vi "Illuminance Correction.vi"(8 "error in (no error)":errorcluster, 11 "Refnum in":T1) -> (0 "error out":errorcluster, 3 "Refnum out":T1)   [LabVIEW 2015]
uses:
  <vilib>/vision/Image Controls.llb/IMAQ Image.ctl
  <vilib>/vision/NI_Vision_Development_Module.lvlib
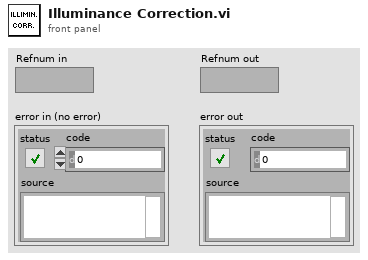
[diagram p1: front panel]
types:
  T1 = typedef "IMAQ Image.ctl" = refnum<image>
  T2 = enum32{"Linear", "Log", "Exp", "Square", "Square root", "Power X", "Power 1/X"}
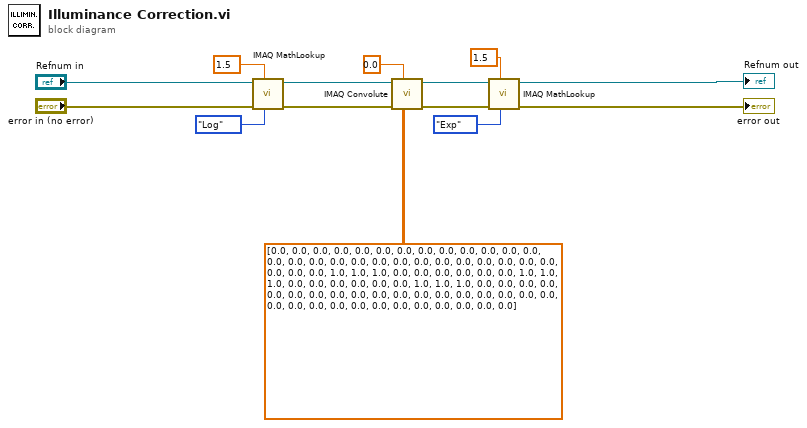
[diagram p0: block diagram]
diagram:
  n1 = call "IMAQ MathLookup"("Operator"=T2."Log", "X Value"=sgl 1.5, "error in (no error)"="error in (no error)", "Image Src"="Refnum in") -> ("error out"=w5:errorcluster, "Image Dst Out"=w7:T1)  [unwired: 3 in, 3 out]
  n2 = call "IMAQ Convolute"("Kernel"=sgl[][] [[0.0, 0.0, 0.0, 0.0, 0.0, 0.0, 0.0, 0.0, 0.0], [0.0, 0.0, 0.0, 0.0, 0.0, 0.0, 0.0, 0.0, 0.0], [0.0, 0.0, 0.0, 0.0, 0.0, 0.0, 0.0, 0.0, 0.0], [0.0, 0.0, 0.0, 1.0, 1.0, 1.0, 0.0, 0.0, 0.0], [0.0, 0.0, 0.0, 1.0, 1.0, 1.0, 0.0, 0.0, 0.0], [0.0, 0.0, 0.0, 1.0, 1.0, 1.0, 0.0, 0.0, 0.0], [0.0, 0.0, 0.0, 0.0, 0.0, 0.0, 0.0, 0.0, 0.0], [0.0, 0.0, 0.0, 0.0, 0.0, 0.0, 0.0, 0.0, 0.0], [0.0, 0.0, 0.0, 0.0, 0.0, 0.0, 0.0, 0.0, 0.0]], "Divider (kernel sum)"=sgl 0.0 ("Divider"), "error in (no error)"=w5, "Image Src"=w7) -> ("error out"=w8:errorcluster, "Image Dst Out"=w12:T1)  [unwired: 3 in, 3 out]
  n3 = call "IMAQ MathLookup"("Operator"=T2."Exp", "X Value"=sgl 1.5, "error in (no error)"=w8, "Image Src"=w12) -> ("error out"=→"error out":errorcluster, "Image Dst Out"=→"Refnum out":T1)  [unwired: 3 in, 3 out]
